vi "Remove Channel.vi"(8 "error in (no error)":errorcluster, 10 "Channel Name":string, 11 "CIFChannelMng in":refnum<class "CIFChannelMng.lvclass">) -> (0 "error out":errorcluster, 3 "CIFChannelMng out":refnum<class "CIFChannelMng.lvclass">)   [LabVIEW 2021, in "CIFChannelMng.lvclass"]
uses:
  CIFChannelMng.lvclass
  CIFChannelMng.lvclass/CIFChannelMng.ctl
  CIFClocks/Typedef/Errors.ctl
  CIFCore/Common/Utilities/Append Error Location.vi
  CIFChannels/CIFChannels.lvclass
  CIFCore/Common/CIFCoreCommon.lvlib
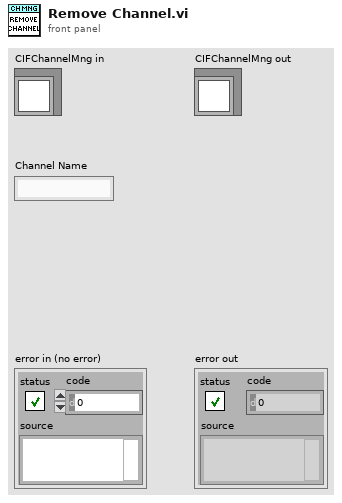
[diagram p1: front panel]
types:
  T1 = typedef "CIFCoreCommon.lvlib/Errors.ctl" = enum16{"Invalid Clock ID", "Long Sleep", "gRPC Server Not Found", "Config Parse", "Timestamp Wrap", "Delayed Execution", "Duplicate Channel", "Missing Channel", "Incorrect Type", "Unregistered Enum"}
  T2 = typedef "CIFChannelMng.lvclass/Channel List for OOB.ctl" = cluster{"Direction":T3, "Type":string, "Custom Config Data":variant, "Connected?":bool, "Connected Name":string}
  T3 = typedef "CIFChannels.lvclass/Direction.ctl" = enum16{"Publisher", "Subscriber"}
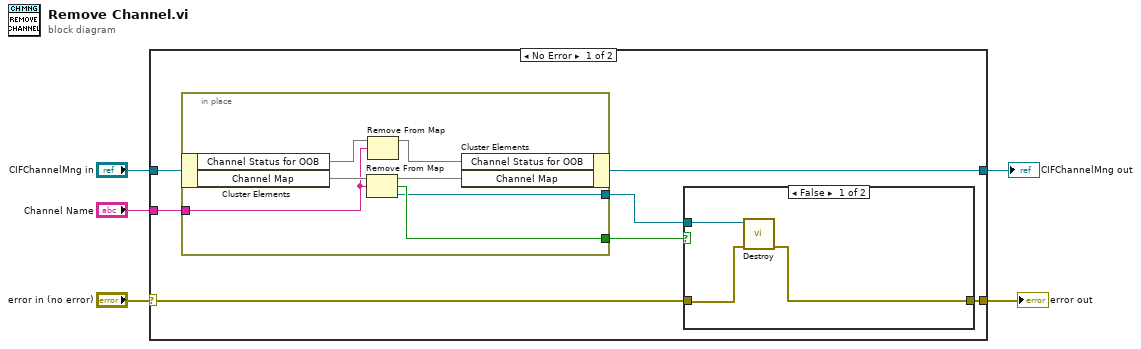
[diagram p0: block diagram]
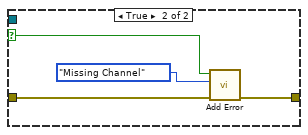
[diagram p2: hidden frame]
diagram:
  n1 = case shown="No Error" "error in (no error)" {
    selector: "error in (no error)" -> [w7 w28]
    tunnel: [w10 w28] -> w5
    tunnel: [w11 w27] -> w4
    tunnel: "CIFChannelMng in" -> [w12 w27]
    tunnel: "Channel Name" -> [w8 _]
    frame No Error {
      n2 = in-place {
        in-place-border: [w26] -> w6
        in-place-border: [w23] -> w9
        in-place-border: w8 -> [w21]
        n3 = in-place-cluster #1(w12) -> ("Channel Status for OOB"=w22:map{string, T2}, "Channel Map"=w25:map{string, refnum<class "CIFChannels.lvclass">})
        n4 = Remove From Map(10:w21, 11:w25) -> (1:w23:refnum<class "CIFChannels.lvclass">, 2:w26:bool, 3:w24:map{string, refnum<class "CIFChannels.lvclass">})
        n5 = Remove From Map(10:w21, 11:w22) -> (3:w20:map{string, T2})  [unwired: 2 out]
        n6 = in-place-cluster #1("Channel Status for OOB"=w20, "Channel Map"=w24) -> (w11:refnum<class "CIFChannelMng.lvclass">)
      }
      n7 = case shown="False" w6 {
        selector: w6 -> [_ w16]
        tunnel: [w13 w18] -> w10
        tunnel: w9 -> [w15 _]
        tunnel: w7 -> [w14 w17]
        frame False {
          n8 = call-dynamic "Destroy.vi"("error in (no error)"=w14, "CIFChannels in"=w15) -> ("error out"=w13:errorcluster)  [unwired: 8 in, 1 out]
        }
        frame True {
          n9 = call "Add Error.vi"("error in (no error)"=w17, "Error"=Errors."Missing Channel", "Insert Error"=w16) -> ("error out"=w18:errorcluster)  [unwired: 8 in]
        }
      }
    }
    frame Error {
    }
  }
  "error out" <- w5
  "CIFChannelMng out" <- w4
